vi "test-PID-tolerance.vi"() -> ()   [LabVIEW 2019]
uses:
  <vilib>/Rock Robotics/WPI/ThirdParty/JAS_Junk/TrajLib/PIDController_NewPeriod.vi
  <vilib>/Rock Robotics/WPI/ThirdParty/JAS_Junk/TrajLib/PIDController_SetTolerancePandV.vi
  <vilib>/Rock Robotics/WPI/ThirdParty/JAS_Junk/TrajLib/ControllerUtil_GetModulusError.vi
  <vilib>/Rock Robotics/SystemInterfaces/NetworkCommunication/NetComm_UsageReport_report.vi
  <vilib>/Rock Robotics/WPI/ThirdParty/JAS_Junk/TrajLib/Util_LibraryGlobals.vi
  <vilib>/Rock Robotics/WPI/ThirdParty/JAS_Junk/TrajLib/Trajectory_Library.lvlib
panel:
  out "T1 -- PV Error 3rd":dbl
  out "T1 - At-SP-False - 3rd":bool
  out "T1 -- PV Error 2nd":dbl
  out "T1 - At-SP-True 2nd":bool
  out "T1 -- PV Error":dbl
  out "T1 - At-SP-False":bool
  out "T0 -- delta PV Error / dT":dbl
  out "T0 -- PV Error":dbl
  out "T0 - At-SP-True":bool
  # "PID Tolerance"
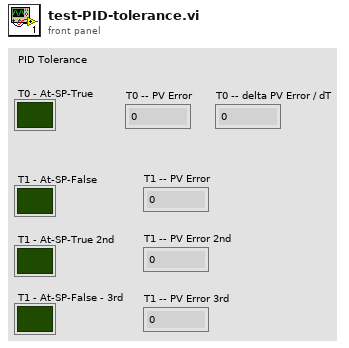
[diagram p1: front panel]
types:
  T1 = typedef "Trajectory_Library.lvlib/PID_CONTROLLER.ctl" = cluster{"Kp":dbl, "Ki":dbl, "Kd":dbl, "Period":dbl, "Max_Integral":dbl, "Min_Integral":dbl, "Max_Input":dbl, "Min_Input":dbl, "Continuous":bool, "PositionError":dbl, "VelocityError":dbl, "PrevError":dbl, "TotalError":dbl, "PositionTolerance":dbl, "VelocityTolerance":dbl, "SetPoint":dbl, "Kf":dbl, "Prev_Deriv":dbl, "Prev_Deriv 2":dbl, "DerivativeFilter":bool, "Min_Output":dbl, "Max_Output":dbl, "Prev_F_P":dbl, "Prev_F_P_2":dbl, "AntiWindupActive":bool, "Measurement":dbl}
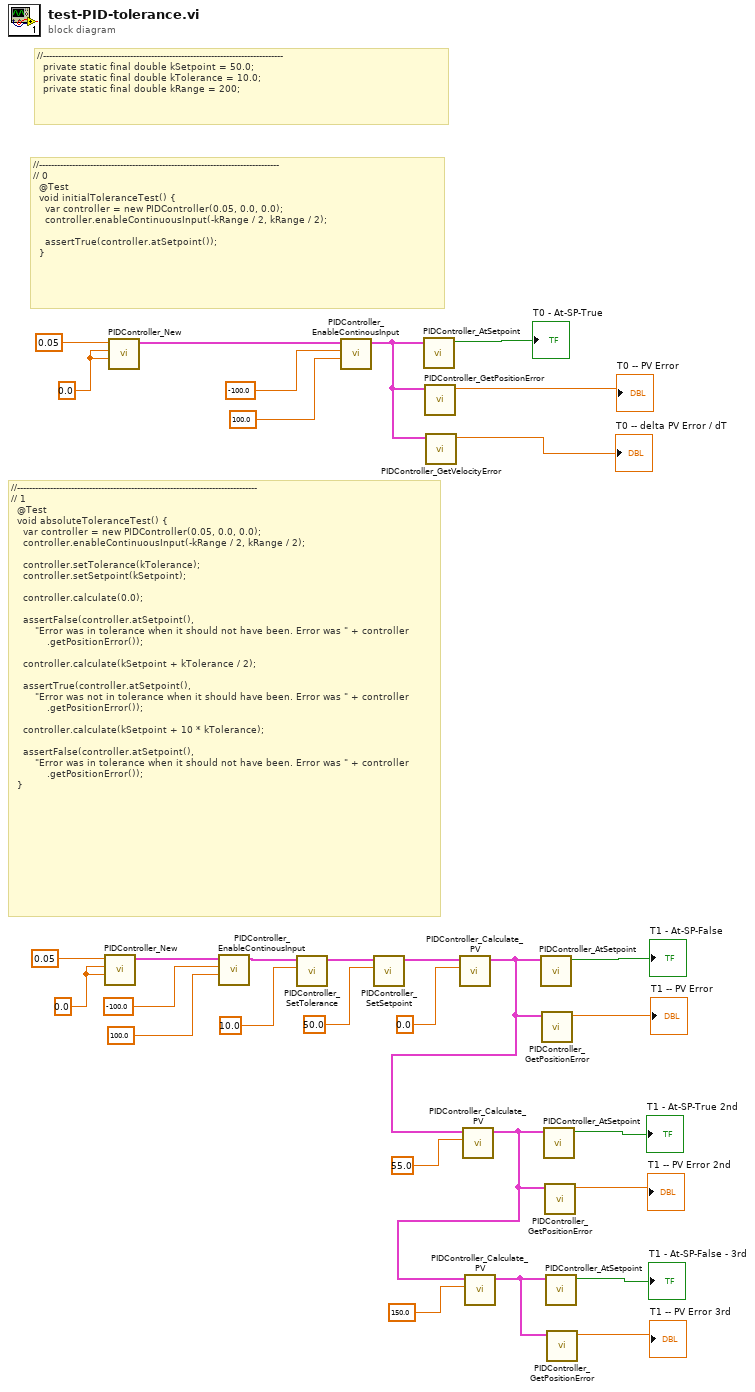
[diagram p0: block diagram]
diagram:
  w22 = 0.0 ("Kp")
  w31 = 0.0 ("Kp")
  # "//--------------------------------------------------------------------------------\n  private static final double kSetpoint = 50.0;\n  private static final double kTolerance = 10.0;\n  private static final double kRange = 200;"
  # "//--------------------------------------------------------------------------------\n// 1\n  @Test\n  void absoluteToleranceTest() {\n    var controller = new PIDController(0.05, 0.0, 0.0);\n    controller.enableContinuousInput(-kRange / 2, kRange / 2);\n\n    controller.setTolerance(kTolerance);\n    controller.setSetpoint(kSetpoint);\n\n    controller.calculate(0.0);\n\n    assertFalse(controller.atSetpoint(),\n        \"Error was in tolerance when it should not have been. Error was \" + controller\n            .getPositionError());\n\n    controller.calculate(kSetpoint + kTolerance / 2);\n\n    assertTrue(controller.atSetpoint(),\n        \"Error was not in tolerance when it should have been. Error was \" + controller\n            .getPositionError());\n\n    controller.calculate(kSetpoint + 10 * kTolerance);\n\n    assertFalse(controller.atSetpoint(),\n        \"Error was in tolerance when it should not have been. Error was \" + controller\n            .getPositionError());\n  }"
  # "//--------------------------------------------------------------------------------\n// 0\n  @Test\n  void initialToleranceTest() {\n    var controller = new PIDController(0.05, 0.0, 0.0);\n    controller.enableContinuousInput(-kRange / 2, kRange / 2);\n\n    assertTrue(controller.atSetpoint());\n  }"
  n1 = call <vilib>:"PIDController_New.vi"("Kd"=w22, "Ki"=w22, "Kp"=0.05) -> ("PID_CONTROLLER"=w18:T1)  [unwired: 8 in]
  n2 = call <vilib>:"PIDController_New.vi"("Kd"=w31, "Ki"=w31, "Kp"=0.05) -> ("PID_CONTROLLER"=w27:T1)  [unwired: 8 in]
  n3 = call <vilib>:"PIDController_EnableContinousInput.vi"("MaxInput"=100.0, "MinInput"=-100.0, "in PID_CONTROLLER"=w18) -> ("out PID_CONTROLLER"=w17:T1)  [unwired: 8 in]
  n4 = call <vilib>:"PIDController_SetTolerance.vi"("PositionTolerance"=10.0, "in PID_CONTROLLER"=w17) -> ("out PID_CONTROLLER"=w15:T1)  [unwired: 9 in]
  n5 = call <vilib>:"PIDController_EnableContinousInput.vi"("MaxInput"=100.0, "MinInput"=-100.0, "in PID_CONTROLLER"=w27) -> ("out PID_CONTROLLER"=w25:T1)  [unwired: 8 in]
  n6 = call <vilib>:"PIDController_SetSetpoint.vi"("Setpoint"=50.0, "in PID_CONTROLLER"=w15) -> ("out PID_CONTROLLER"=w13:T1)  [unwired: 9 in]
  n7 = call <vilib>:"PIDController_AtSetpoint.vi"("in PID_CONTROLLER"=w25) -> ("AtSetpoint"=→"T0 - At-SP-True":bool)  [unwired: 10 in]
  n8 = call <vilib>:"PIDController_GetPositionError.vi"("in PID_CONTROLLER"=w25) -> ("PositionError"=→"T0 -- PV Error":dbl)  [unwired: 10 in]
  n9 = call <vilib>:"PIDController_GetVelocityError.vi"("in PID_CONTROLLER"=w25) -> ("VelocityError"=→"T0 -- delta PV Error / dT":dbl)  [unwired: 10 in]
  n10 = call <vilib>:"PIDController_Calculate_PV.vi"("PV"=0.0, "in PID_CONTROLLER"=w13) -> ("out PID_CONTROLLER"=w8:T1)  [unwired: 8 in, 1 out]
  n11 = call <vilib>:"PIDController_Calculate_PV.vi"("PV"=55.0, "in PID_CONTROLLER"=w8) -> ("out PID_CONTROLLER"=w1:T1)  [unwired: 8 in, 1 out]
  n12 = call <vilib>:"PIDController_Calculate_PV.vi"("PV"=150.0, "in PID_CONTROLLER"=w1) -> ("out PID_CONTROLLER"=w4:T1)  [unwired: 8 in, 1 out]
  n13 = call <vilib>:"PIDController_AtSetpoint.vi"("in PID_CONTROLLER"=w8) -> ("AtSetpoint"=→"T1 - At-SP-False":bool)  [unwired: 10 in]
  n14 = call <vilib>:"PIDController_GetPositionError.vi"("in PID_CONTROLLER"=w8) -> ("PositionError"=→"T1 -- PV Error":dbl)  [unwired: 10 in]
  n15 = call <vilib>:"PIDController_AtSetpoint.vi"("in PID_CONTROLLER"=w1) -> ("AtSetpoint"=→"T1 - At-SP-True 2nd":bool)  [unwired: 10 in]
  n16 = call <vilib>:"PIDController_GetPositionError.vi"("in PID_CONTROLLER"=w1) -> ("PositionError"=→"T1 -- PV Error 2nd":dbl)  [unwired: 10 in]
  n17 = call <vilib>:"PIDController_AtSetpoint.vi"("in PID_CONTROLLER"=w4) -> ("AtSetpoint"=→"T1 - At-SP-False - 3rd":bool)  [unwired: 10 in]
  n18 = call <vilib>:"PIDController_GetPositionError.vi"("in PID_CONTROLLER"=w4) -> ("PositionError"=→"T1 -- PV Error 3rd":dbl)  [unwired: 10 in]
